vi "GET_Text.vi"(8 "error in (no error)":errorcluster {"code" min=0 max=0}, 11 "Settings.lvclass in":refnum<class "Settings.lvclass">) -> (0 "error out":errorcluster {"code" min=0 max=0}, 2 "Text":cluster{"Font":T1, "Alignment":T2, "Size":T3}={"Font"="", "Alignment"=0, "Size"=3} {"Alignment" items=["left", "center", "right"]}, 3 "Settings.lvclass out":refnum<class "Settings.lvclass">)   [LabVIEW 2020, in "Settings.lvclass"]
uses:
  Settings.lvclass
  Settings.lvclass/Settings.ctl
  vi.lib/LabVIEW Icon API/lv_icon/Controls/Font.ctl
  Controls/Font Size.ctl
  vi.lib/LabVIEW Icon API/lv_icon/Controls/Alignment.ctl
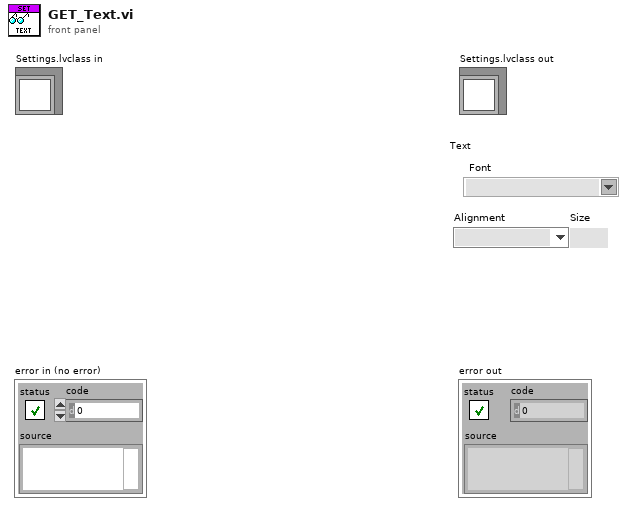
[diagram p1: front panel]
types:
  T1 = typedef "Font.ctl" = string
  T2 = typedef "Alignment.ctl" = u16
  T3 = typedef "Font Size.ctl" = u8
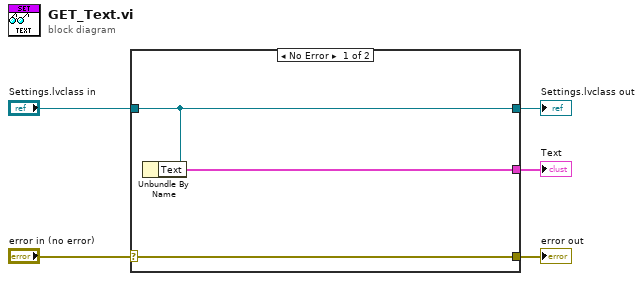
[diagram p0: block diagram]
diagram:
  n1 = case shown="No Error" "error in (no error)" {
    selector: "error in (no error)" -> [w8 w9]
    tunnel: [w8 w9] -> w4
    tunnel: [w7 w10] -> w2
    tunnel: "Settings.lvclass in" -> [w7 w10]
    tunnel: [w6 _] -> w1
    frame No Error {
      n2 = Unbundle By Name(w7) -> ("Text"=w6:cluster{"Font":T1, "Alignment":T2, "Size":T3})
    }
    frame Error {
    }
  }
  "error out" <- w4
  "Settings.lvclass out" <- w2
  "Text" <- w1
